vi "Write Parameters.vi"(10 "Parameters":u32[](array[numeric])=[300, 180000, 300, 5000, 180000, 3000], 11 "valve_VCH_ZM_state in":refnum<class "HE_ZM_state.lvclass">) -> (3 "valve_VCH_ZM_state out":refnum<class "HE_ZM_state.lvclass">)   [LabVIEW 2019, in "Heating.lvlib" / "HE_ZM_state.lvclass"]
uses:
  HE_ZM_state.lvclass
  HE_ZM_state.lvclass/HE_ZM_state.ctl
panel:
  # "T_start_delay\nT_heat_start\nT_stop_delay\nT_set_min\nT_heat_stop\nT_restart_delay"
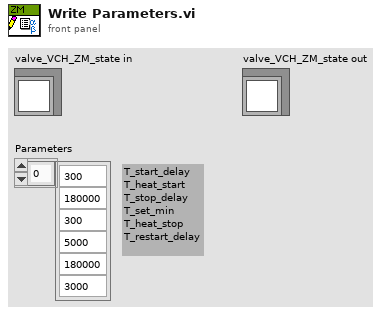
[diagram p1: front panel]
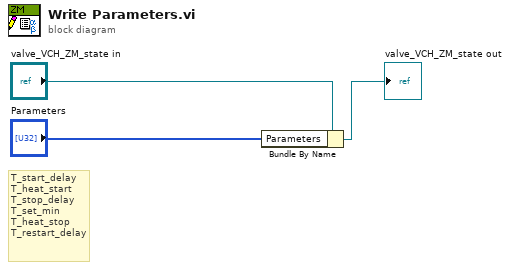
[diagram p0: block diagram]
diagram:
  # "T_start_delay\nT_heat_start\nT_stop_delay\nT_set_min\nT_heat_stop\nT_restart_delay"
  n1 = Bundle By Name(cluster="valve_VCH_ZM_state in", "Parameters"="Parameters") -> (→"valve_VCH_ZM_state out":refnum<class "HE_ZM_state.lvclass">)
